vi "SubscribeMethods.vi"   [LabVIEW 2014]
uses:
  EmergancyController_class/EmergancyController.lvclass
  XmlLogger_class/XmlLogger.lvclass
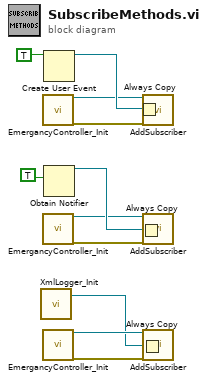
[diagram p0: block diagram]
diagram:
  n1 = call "XmlLogger_Init.vi"() -> ("object out"=w2:refnum<class "XmlLogger.lvclass">)  [unwired: 18 in, 1 out]
  n2 = call "EmergancyController_Init.vi"() -> ("object out"=w9:refnum<class "EmergancyController.lvclass">, "error out"=w8:errorcluster)  [unwired: 18 in]
  n3 = call "EmergancyController_Init.vi"() -> ("object out"=w5:refnum<class "EmergancyController.lvclass">, "error out"=w4:errorcluster)  [unwired: 18 in]
  n4 = call "EmergancyController_Init.vi"() -> ("object out"=w3:refnum<class "EmergancyController.lvclass">, "error out"=w1:errorcluster)  [unwired: 18 in]
  n5 = Create User Event(user event datatype=TRUE) -> (user event=w10:refnum<user-event>)  [unwired: 1 in, 1 out]
  n6 = Obtain Notifier(notification data type=TRUE) -> (notifier out=w6:refnum<notifier>)  [unwired: 3 in, 2 out]
  n7 = Always Copy(1:w10) -> ()  [unwired: 1 out]
  n8 = Always Copy(1:w6) -> ()  [unwired: 1 out]
  n9 = Always Copy(1:w2) -> ()  [unwired: 1 out]
  n10 = call-dynamic "AddSubscriber.vi"("object in"=w9, "error in (no error)"=w8) -> ()  [unwired: 16 in, 2 out]
  n11 = call-dynamic "AddSubscriber.vi"("object in"=w5, "error in (no error)"=w4) -> ()  [unwired: 16 in, 2 out]
  n12 = call-dynamic "AddSubscriber.vi"("object in"=w3, "error in (no error)"=w1) -> ()  [unwired: 16 in, 2 out]
